vi "lamp-start.vi"(8 "error in (no error)":errorcluster, 10 "Set":bool, 11 "Lamp":refnum<vi>) -> (0 "error out":errorcluster)   [LabVIEW 2016]
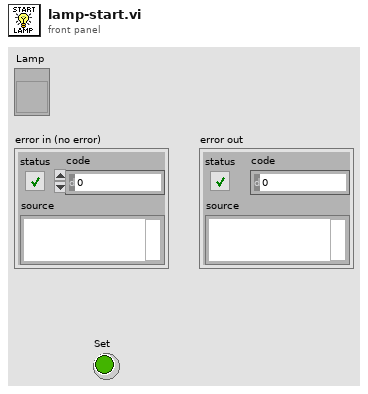
[diagram p1: front panel]
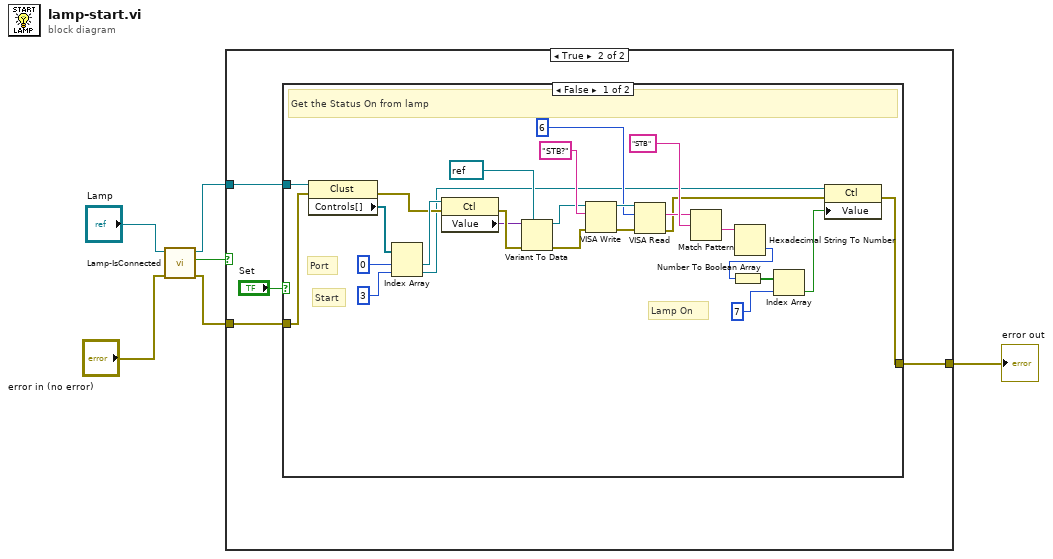
[diagram p0: block diagram]
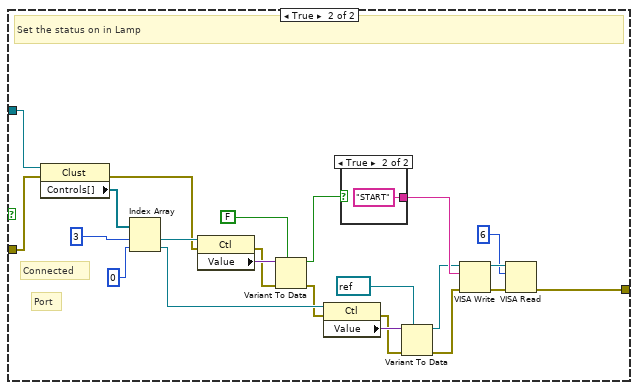
[diagram p3: hidden frame]
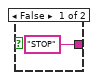
[diagram p4: hidden frame]
diagram:
  n1 = call "Lamp-IsConnected.vi"("error in (no error)"="error in (no error)", "Lamp in"="Lamp") -> ("error out"=w3:errorcluster, "Connected"=w1:bool, "Lamp out"=w2:refnum<vi>)  [unwired: 7 in]
  n2 = case shown="True" w1 {
    tunnel: [w7 w11] -> w6
    tunnel: w3 -> [w7 w9]
    tunnel: w2 -> [_ w8]
    frame False {
    }
    frame True {
      n3 = case shown="False" "Set" {
        tunnel: [w25 w58] -> w11
        tunnel: w9 -> [w32 w52]
        tunnel: w8 -> [w33 w53]
        frame False {
          # "Lamp On"
          # "Start"
          # "Port"
          # "Get the Status On from lamp"
          n4 = property class="Clust"(reference=w33, error in=w32) -> (error out=w20:errorcluster, "Controls[]"=w23:refnum<vi>[])  [unwired: 1 out]
          n5 = Index Array(array=w23, index #1=0 ("index"), index #2=3 ("index")) -> (element #1=w21:refnum<vi>, element #2=w14:refnum<vi>)
          n6 = property class="Ctl"(reference=w21, error in=w20) -> (error out=w19:errorcluster, "Value"=w18:variant)  [unwired: 1 out]
          n7 = Variant To Data(error in=w19, type=refnum<visa-resource-name> refnum ("reference out"), Variant=w18) -> (data=w16:refnum<visa-resource-name>, error out=w26:errorcluster)
          n8 = VISA Write(VISA resource name=w16, write buffer="STB?", error in (no error)=w26) -> (VISA resource name out=w30:refnum<visa-resource-name>, error out=w29:errorcluster)  [unwired: 1 out]
          n9 = VISA Read(VISA resource name=w30, byte count=u32 6, error in (no error)=w29) -> (read buffer=w27:string, error out=w12:errorcluster)  [unwired: 2 out]
          n10 = Match Pattern(string=w27, regular expression="STB") -> (after substring=w36:string)  [unwired: 1 in, 3 out]
          n11 = Hexadecimal String To Number(string=w36) -> (number=w24:u32)  [unwired: 2 in, 1 out]
          n12 = Number To Boolean Array(number=w24) -> (Boolean array=w35:bool[])
          n13 = Index Array(array=w35, index=7) -> (element=w13:bool)
          n14 = property class="Ctl"(reference=w14, error in=w12, "Value"=w13) -> (error out=w25:errorcluster)  [unwired: 1 out]
        }
        frame True {
          # "Port"
          # "Connected"
          # "Set the status on in Lamp"
          n15 = property class="Clust"(reference=w53, error in=w52) -> (error out=w50:errorcluster, "Controls[]"=w54:refnum<vi>[])  [unwired: 1 out]
          n16 = Index Array(array=w54, index #1=3 ("index"), index #2=0 ("index")) -> (element #1=w51:refnum<vi>, element #2=w44:refnum<vi>)
          n17 = property class="Ctl"(reference=w51, error in=w50) -> (error out=w48:errorcluster, "Value"=w49:variant)  [unwired: 1 out]
          n18 = Variant To Data(error in=w48, type=FALSE, Variant=w49) -> (data=w45:bool, error out=w43:errorcluster)
          n19 = property class="Ctl"(reference=w44, error in=w43) -> (error out=w41:errorcluster, "Value"=w42:variant)  [unwired: 1 out]
          n20 = case shown="True" w45 {
            tunnel: ["STOP" "START"] -> w60
            frame False {
            }
            frame True {
            }
          }
          n21 = Variant To Data(error in=w41, type=refnum<visa-resource-name> refnum ("reference out"), Variant=w42) -> (data=w39:refnum<visa-resource-name>, error out=w38:errorcluster)
          n22 = VISA Write(VISA resource name=w39, write buffer=w60, error in (no error)=w38) -> (VISA resource name out=w57:refnum<visa-resource-name>, error out=w59:errorcluster)  [unwired: 1 out]
          n23 = VISA Read(VISA resource name=w57, byte count=6, error in (no error)=w59) -> (error out=w58:errorcluster)  [unwired: 3 out]
        }
      }
    }
  }
  "error out" <- w6
